vi "CalcArmPressure.vi"(8 "error in (no error)":errorcluster, 11 "Armpres":dbl[][](array[numeric])) -> (0 "error out":errorcluster, 2 "Method":dbl, 3 "Array Out":dbl[](array[numeric]))   [LabVIEW 2013, in "main.lvlib"]
uses:
  main.lvlib
  Controls/Enum Variables.ctl
  <vilib>/Analysis/NI_AALBase.lvlib
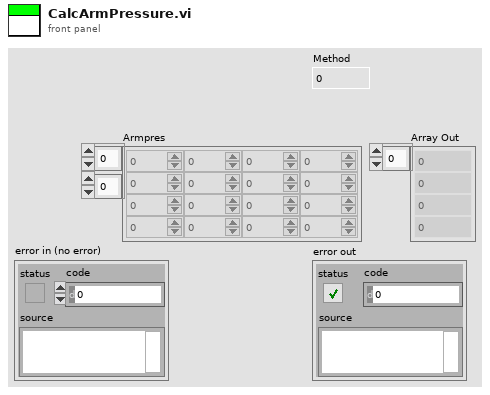
[diagram p1: front panel]
types:
  T1 = typedef "main.lvlib/Enum Variables.ctl" = enum16{"SetAcqFilter", "GetAcqFilter", "Set Filter", "Get Filter", "Set Height", "Get Height", "Set Recorded Height", "Get Recorded Height", "Set Blue Pressure", "Get Blue Pressure", "Set Red Pressure", "Get Red Pressure", "Init", "Reset Pressure", "Set Red Cursors", "Get Red Cursors", "Set Blue Cursors", "Get Blue Cursors", "Set Language", "Get Language", "Set Active Graphs", "Get ActiveGraphs", "Set Method", "Get Method", "Set Encryption", "Get Encryption", "Set ExcelVersion", "Get ExcelVersion", "Set DICOM Avail", "Get DICOM Avail", "Set DICOM Encode", "Get DICOM Encode", "Set JournalExport", "Get JournalExport", "Set Sequence", "Get Sequence", "Set DAQ Connected", "Get DAQ Connected", "Set Current Graph", "Get Current Graph", "Set General Settings", "Get Hyphenation", "Set Arm Calc Method", "Get Arm Calc Method", "Set Dicom Tags", "Get Dicom Tags", "Set BT Serial", "Get BT Serial", "Set BT Accepted Serials", "Get BT Accepted Serials", "Get BT License", "Set BT License"}
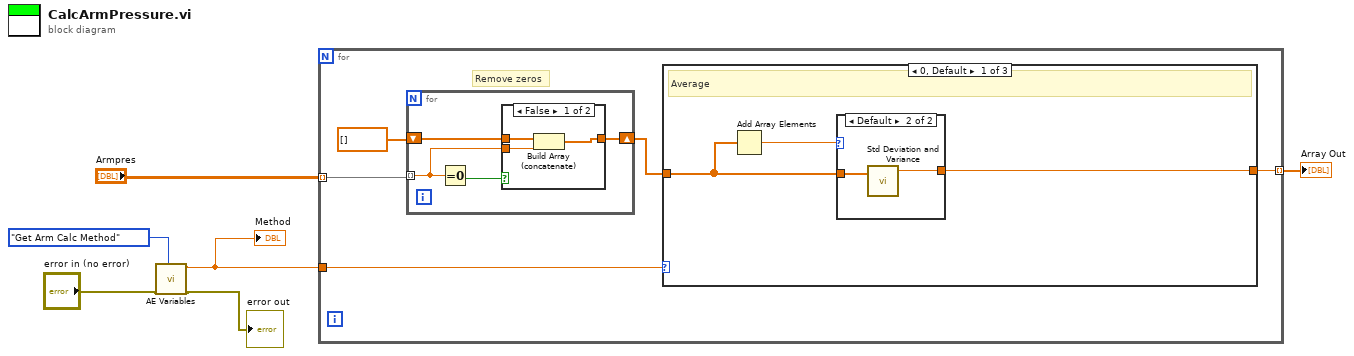
[diagram p0: block diagram]
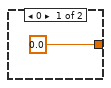
[diagram p3: hidden frame]
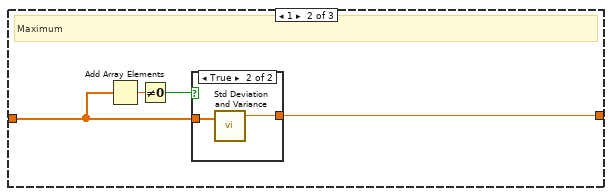
[diagram p4: hidden frame]
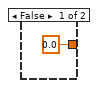
[diagram p5: hidden frame]
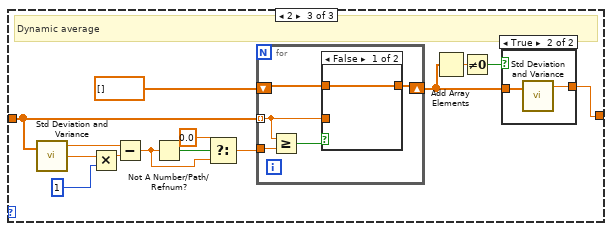
[diagram p6: hidden frame]
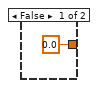
[diagram p7: hidden frame]
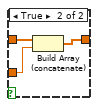
[diagram p8: hidden frame]
diagram:
  n1 = call "AE Variables.vi"("error in (no error)"="error in (no error)", "Action"=Enum_Variables."Get Arm Calc Method") -> ("NumericOut"=w1:dbl, "error out"=→"error out":errorcluster)  [unwired: 10 in, 6 out]
  "Method" <- w1
  n2 = for {
    tunnel: "Armpres" -> [w8] mode=indexing
    tunnel: w1 -> [w11]
    tunnel: [w10] -> w5 mode=indexing
    # "Remove zeros"
    n3 = for {
      shift-right: [w15] -> w7
      shift-left: dbl[] [] -> [w13]
      tunnel: w8 -> [w12] mode=indexing
      n4 = Equal To 0?(x=w12) -> (x = 0?=w14:bool)
      n5 = case shown="False" w14 {
        tunnel: [w18 w19] -> w15
        tunnel: w13 -> [w17 w19]
        tunnel: w12 -> [w16 _]
        frame False {
          n6 = Build Array (concatenate)(w17, w16) -> (w18:dbl[])
        }
        frame True {
        }
      }
    }
    n7 = case shown="0, Default" w11 {
      tunnel: w7 -> [w21 w28 w45]
      tunnel: [w22 w29 w43] -> w10
      frame 0, Default {
        # "Average"
        n8 = Add Array Elements(numeric array=w21) -> (sum=w20:dbl)
        n9 = case shown="Default" w20 {
          tunnel: [0.0 w24] -> w22
          tunnel: w21 -> [_ w25]
          frame 0 {
          }
          frame Default {
            n10 = call <vilib>:"Std Deviation and Variance.vi"("X"=w25) -> ("mean"=w24:dbl)  [unwired: 1 in, 2 out]
          }
        }
      }
      frame 1 {
        # "Maximum"
        n11 = Add Array Elements(numeric array=w28) -> (sum=w27:dbl)
        n12 = Not Equal To 0?(x=w27) -> (x != 0?=w26:bool)
        n13 = case shown="True" w26 {
          tunnel: [0.0 ("mean") w32] -> w29
          tunnel: w28 -> [_ w31]
          frame False {
          }
          frame True {
            n14 = call <vilib>:"Std Deviation and Variance.vi"("X"=w31) -> ("mean"=w32:dbl)  [unwired: 1 in, 2 out]
          }
        }
      }
      frame 2 {
        # "Dynamic average"
        n15 = call <vilib>:"Std Deviation and Variance.vi"("X"=w45) -> ("mean"=w44:dbl, "standard deviation"=w42:dbl)  [unwired: 1 in, 1 out]
        n16 = Multiply(x=w42, y=1) -> (x*y=w41:dbl)
        n17 = Subtract(x=w44, y=w41) -> (x-y=w34:dbl)
        n18 = Not A Number/Path/Refnum?(number/path/refnum=w34) -> (NaN/Path/Refnum?=w35:bool)
        n19 = Select(t=0.0, s=w35, f=w34) -> (s? t:f=w36:dbl)
        n20 = for {
          shift-right: [w51] -> w39
          shift-left: dbl[] [] -> [w52]
          tunnel: w45 -> [w50] mode=indexing
          tunnel: w36 -> [w54]
          n21 = Greater Or Equal?(x=w50, y=w54) -> (x >= y?=w53:bool)
          n22 = case shown="False" w53 {
            tunnel: w52 -> [w55 w58]
            tunnel: [w55 w57] -> w51
            tunnel: w50 -> [_ w56]
            frame False {
            }
            frame True {
              n23 = Build Array (concatenate)(w58, w56) -> (w57:dbl[])
            }
          }
        }
        n24 = Add Array Elements(numeric array=w39) -> (sum=w38:dbl)
        n25 = Not Equal To 0?(x=w38) -> (x != 0?=w37:bool)
        n26 = case shown="True" w37 {
          tunnel: [0.0 ("mean") w49] -> w43
          tunnel: w39 -> [_ w48]
          frame False {
          }
          frame True {
            n27 = call <vilib>:"Std Deviation and Variance.vi"("X"=w48) -> ("mean"=w49:dbl)  [unwired: 1 in, 2 out]
          }
        }
      }
    }
  }
  "Array Out" <- w5
